vi "Read Diagnotics interval.vi"(8 "error in (no error)":errorcluster, 11 "Instrument Actor in":refnum<class "Instrument Actor.lvclass">) -> (0 "error out":errorcluster, 2 "Diagnotics interval":dbl=1.0, 3 "Instrument Actor out":refnum<class "Instrument Actor.lvclass">)   [LabVIEW 2024, in "Instrument Actor.lvclass"]
uses:
  Instrument Actor.lvclass
  Instrument Actor.lvclass/Instrument Actor.ctl
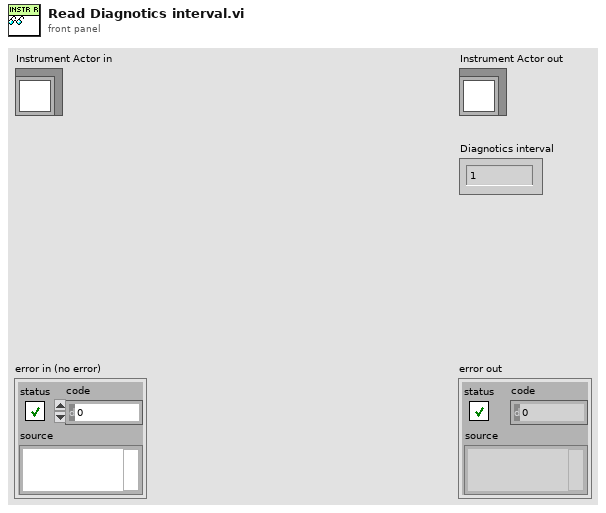
[diagram p1: front panel]
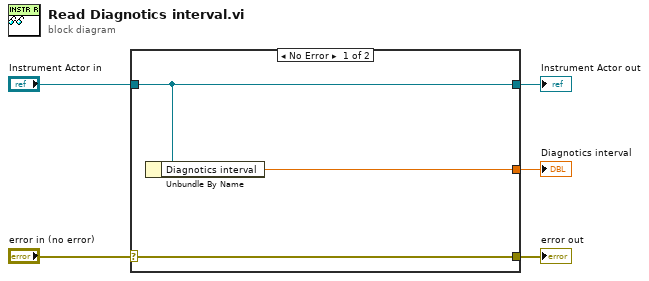
[diagram p0: block diagram]
diagram:
  n1 = case shown="No Error" "error in (no error)" {
    selector: "error in (no error)" -> [w8 w9]
    tunnel: [w8 w9] -> w4
    tunnel: [w7 w10] -> w2
    tunnel: "Instrument Actor in" -> [w7 w10]
    tunnel: [w6 _] -> w1
    frame No Error {
      n2 = Unbundle By Name(w7) -> ("Diagnotics interval"=w6:dbl)
    }
    frame Error {
    }
  }
  "error out" <- w4
  "Instrument Actor out" <- w2
  "Diagnotics interval" <- w1
